vi "FTW-ActorTemplate.vi"(0 "FTW Actor Instance Configuration":string="{\n  \"Identity\": \"ActorName\",\n  \"InboxAddress\": \"inproc://*\",\n  \"PublisherAddress\": \"\",\n  \"LoggerAddress\": \"\",\n  \"DebugEnableInboxLogging\": false,\n  \"DebugEnableJobLogging\": false,\n  \"LauncherAddress\": \"\"\n}", 11 "ErrorIn":errorcluster) -> (15 "Error":errorcluster)   [LabVIEW 2013]
uses:
  src/Instance/FTW-ActorInstance.lvclass
  src/Message/Base/FTW-Message.lvclass
  src/Instance/FTW-ActorInstance.lvclass/FTW-ActorInstance.ctl
  src/JobSequencer/FTW-SEQ-Current.vi
  src/Message/Request/FTW-Message-IncomingRequest.lvclass
panel:
  # "Inputs"
  # "Outputs"
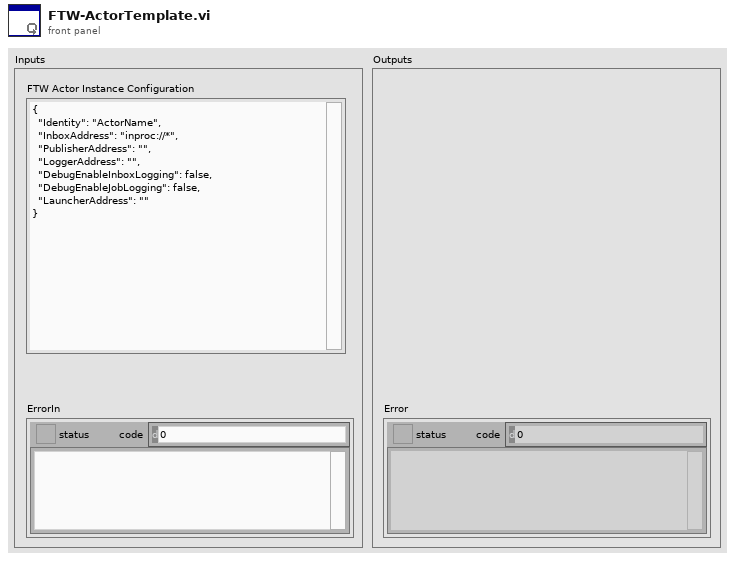
[diagram p1: front panel]
types:
  T1 = cluster{"Incoming Requests":refnum<event-registration>, "Local Messages":refnum<event-registration>, "Additional Registration Types":refnum<event-registration>}
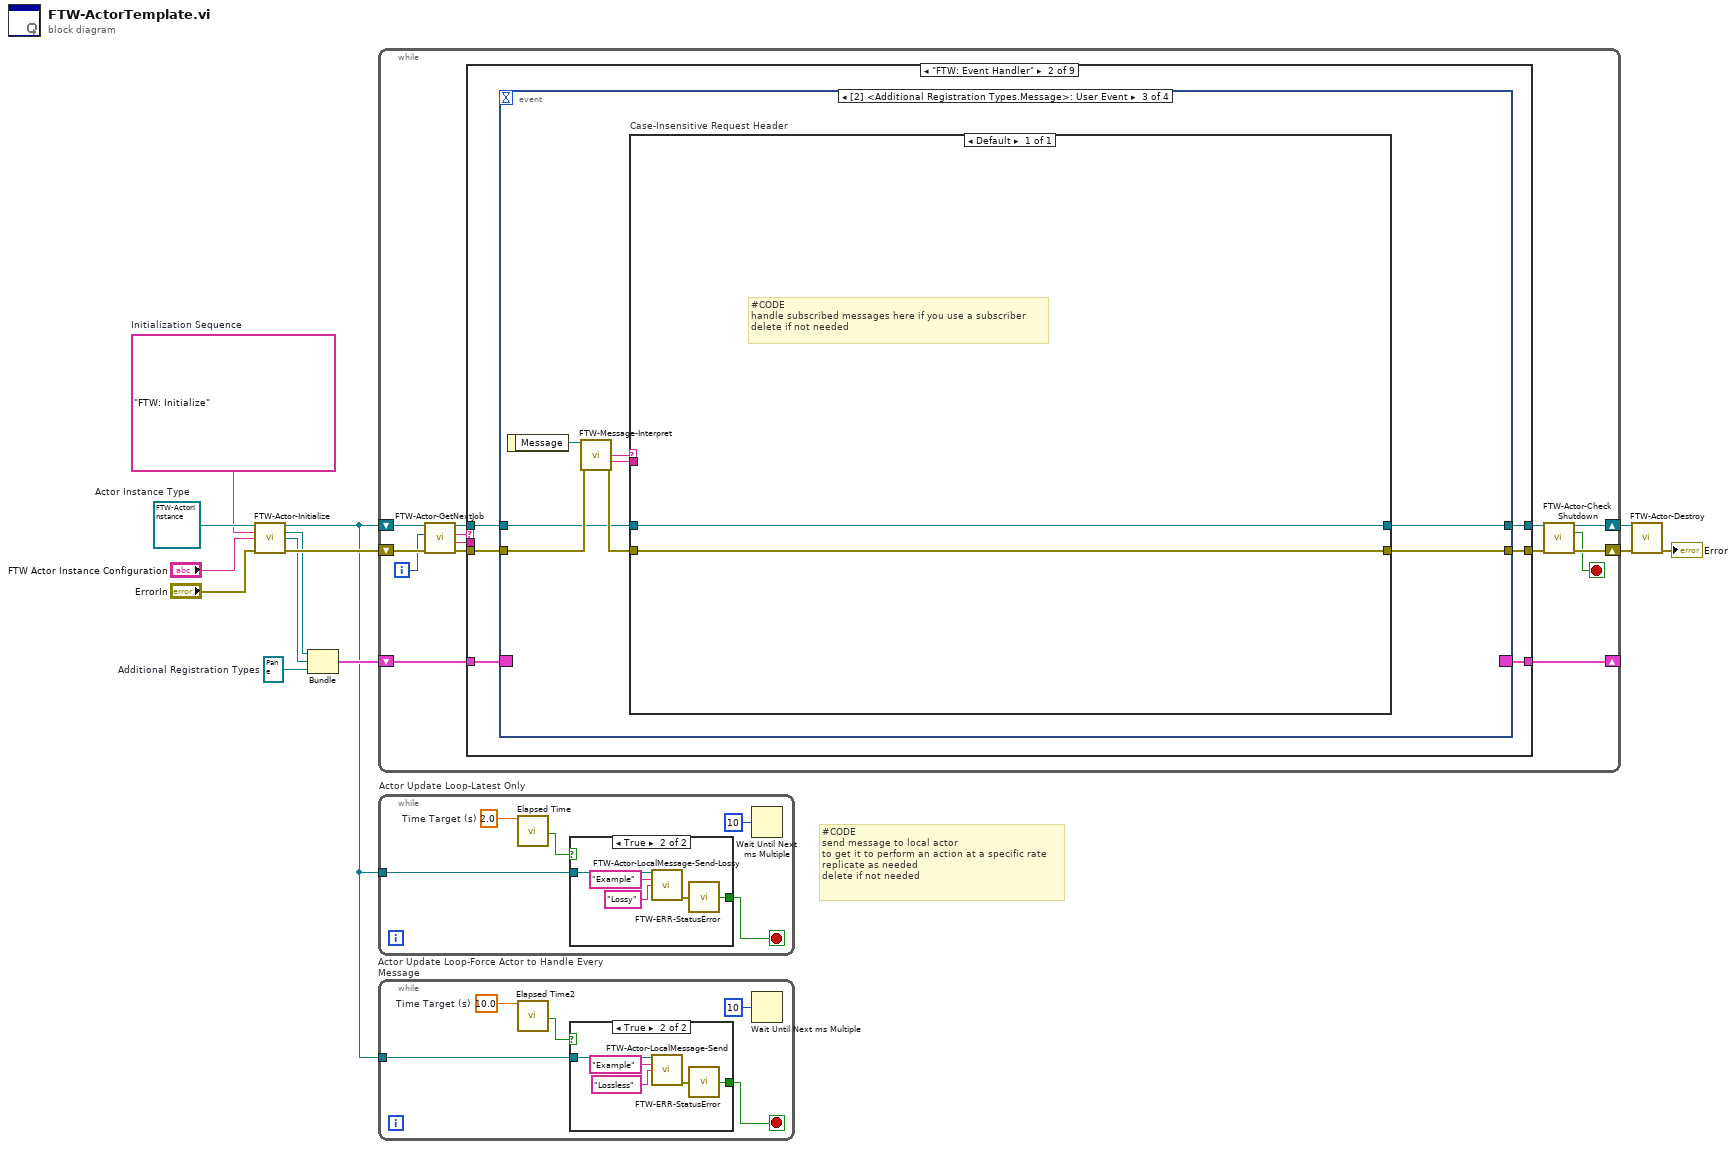
[diagram p0: block diagram]
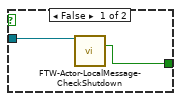
[diagram p2: hidden frame]
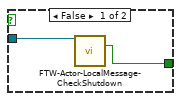
[diagram p3: hidden frame]
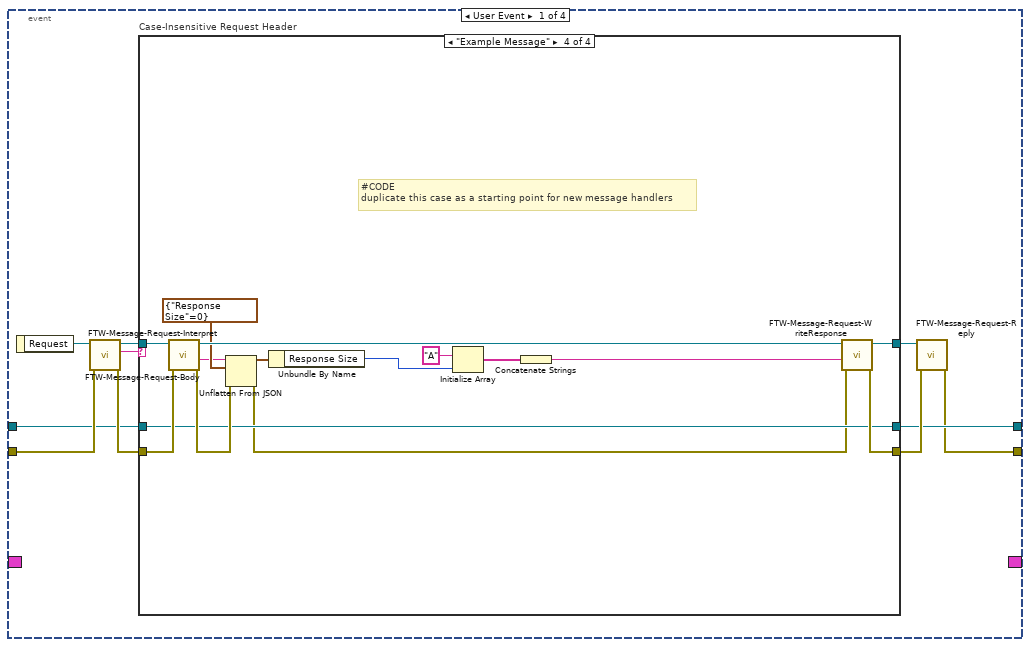
[diagram p5: hidden frame]
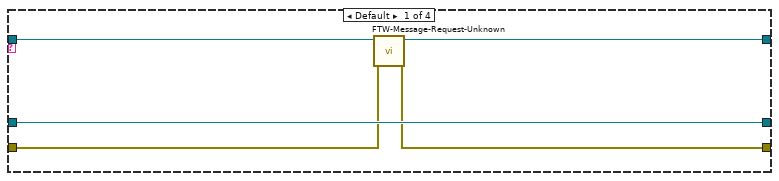
[diagram p6: hidden frame]
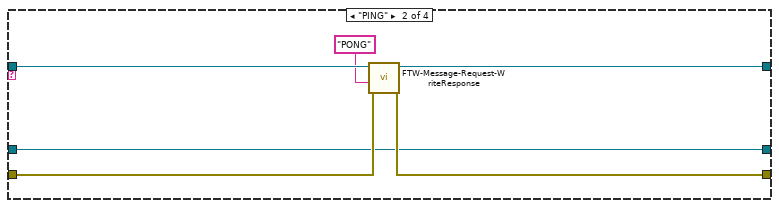
[diagram p7: hidden frame]
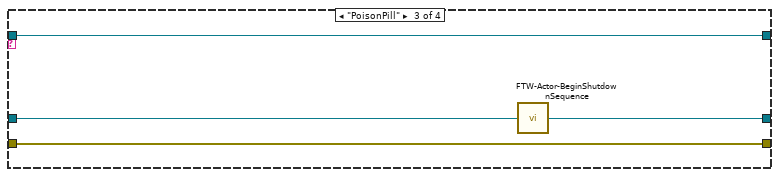
[diagram p8: hidden frame]
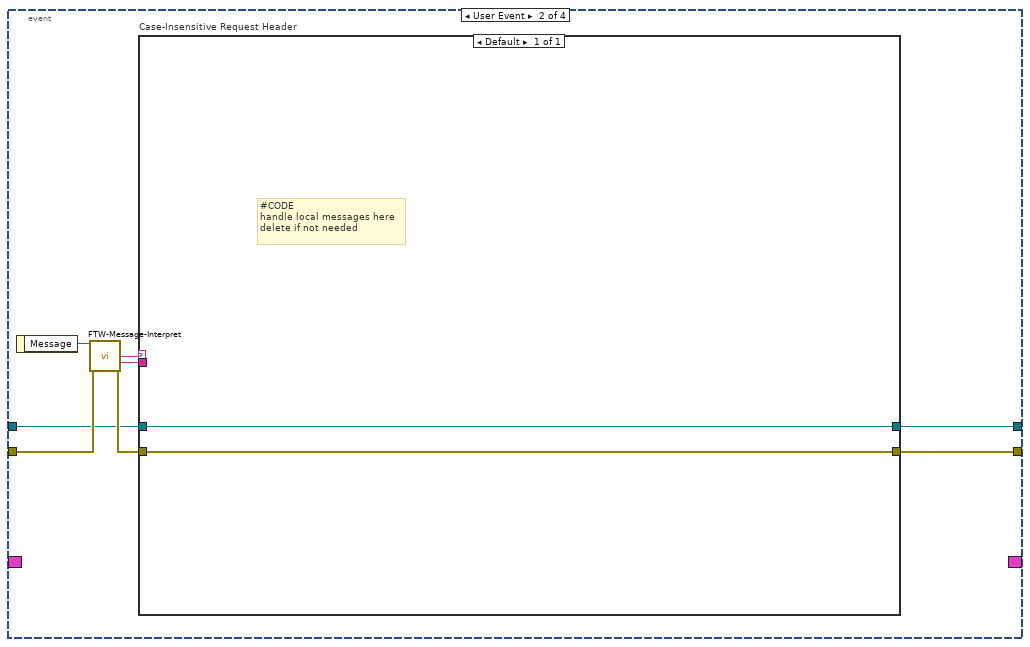
[diagram p9: hidden frame]
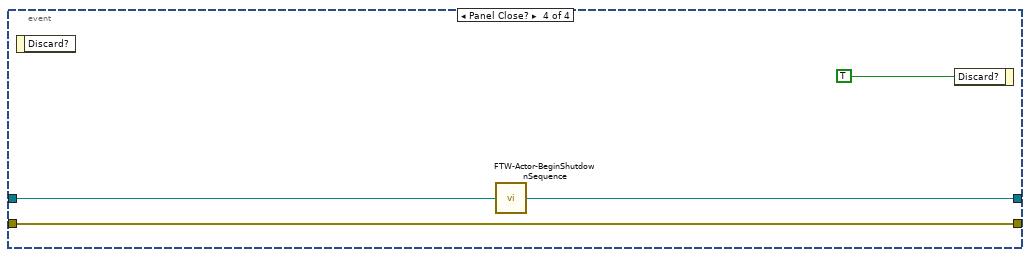
[diagram p10: hidden frame]
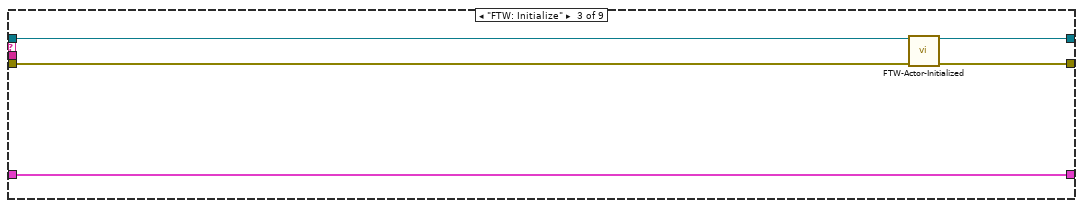
[diagram p11: hidden frame]
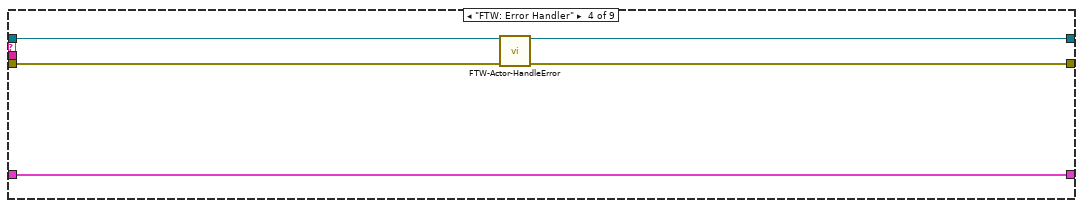
[diagram p12: hidden frame]
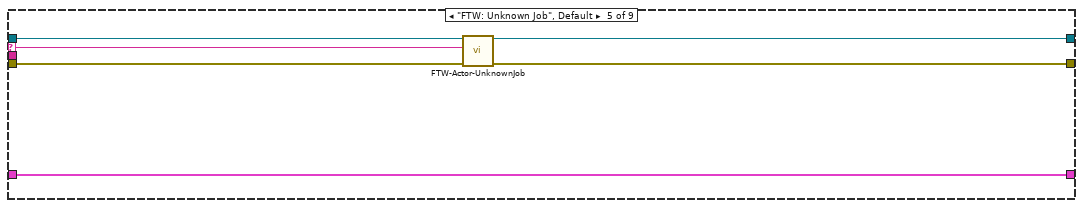
[diagram p13: hidden frame]
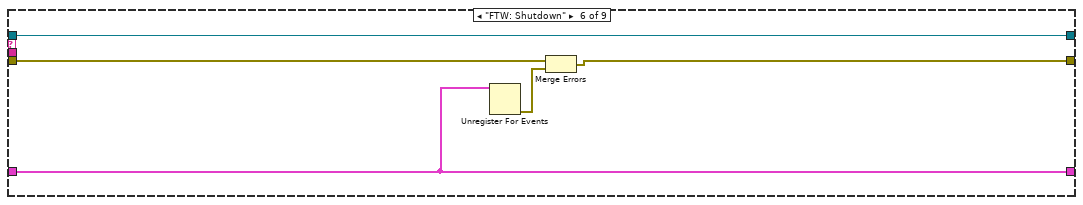
[diagram p14: hidden frame]
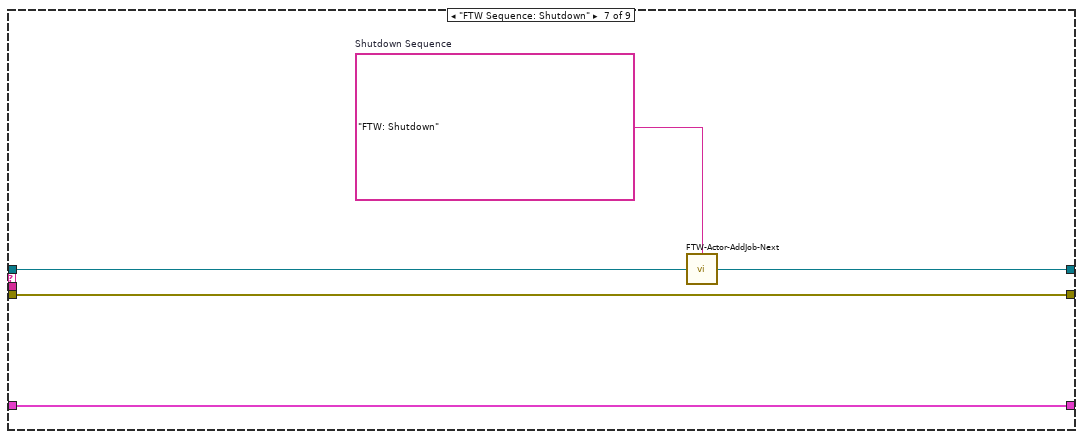
[diagram p15: hidden frame]
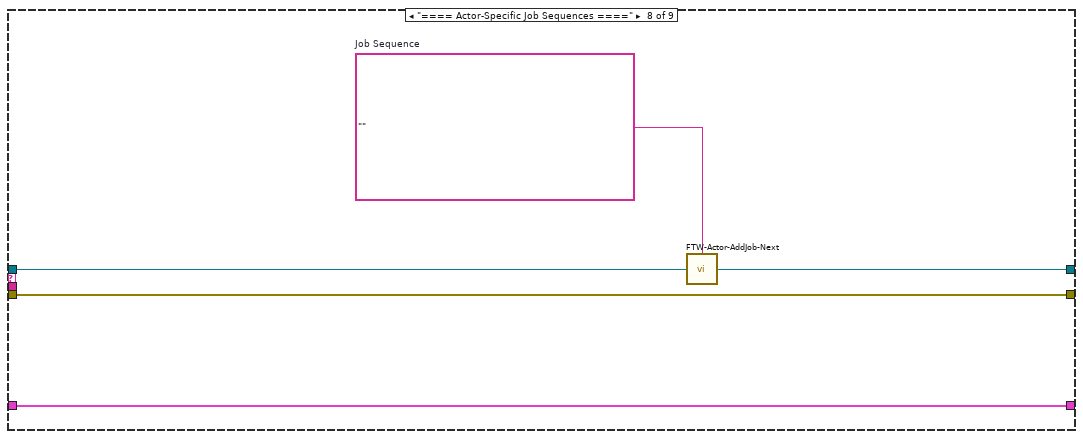
[diagram p16: hidden frame]
diagram:
  w1 = refnum<event-registration> refnum  # Additional Registration Types
  w9 = refnum<class "FTW-ActorInstance.lvclass"> refnum  # Actor Instance Type
  w8 = "FTW: Initialize"  # Initialization Sequence
  # "#CODE\nsend message to local actor\nto get it to perform an action at a specific rate\nreplicate as needed\ndelete if not needed"
  n1 = call-dynamic "FTW-Actor-Initialize.vi"("FTW Actor Instance Type"=w9, "Initialization Job Sequence"=w8, "Actor Instance Configuration"="FTW Actor Instance Configuration", "error in"="ErrorIn") -> ("FTW Actor Instance"=w2:refnum<class "FTW-ActorInstance.lvclass">, "Incoming Requests"=w4:refnum<event-registration>, "Local Messages"=w3:refnum<event-registration>, "error out"=w10:errorcluster)  [unwired: 8 in]
  n2 = Bundle("Incoming Requests"=w4, "Local Messages"=w3, "Additional Registration Types"=w1) -> (w6:T1)  [unwired: 1 in]
  n3 = while {
    shift-right: [w17] -> w12
    shift-left: w10 -> [w24]
    shift-right: [w14] -> _
    shift-left: w6 -> [w27]
    shift-right: [w19] -> w13
    shift-left: w2 -> [w26]
    i -> [w15]
    stop <- w16 stop-if-true
    n4 = call "FTW-Actor-GetNextJob.vi"("error in"=w24, "Jobs Performed"=w15, "FTW Actor Instance"=w26) -> ("error out"=w23:errorcluster, "Job Data"=w21:string, "Job Name"=w22:string, "FTW Actor Instance out"=w25:refnum<class "FTW-ActorInstance.lvclass">)  [unwired: 5 in]
    n5 = case shown="\"FTW: Event Handler\"" w22 {
      selector: w22 -> [_ _ _ _ w111 _ _ _ _]
      tunnel: [w29 w36 w101 w106 w114 w120 w125 w130 w134] -> w18
      tunnel: w23 -> [w29 w35 w104 w108 w115 w121 w125 w130 w134]
      tunnel: w27 -> [w30 w31 w105 w110 w116 w117 w126 w131 w133]
      tunnel: [w30 w34 w105 w110 w116 w117 w126 w131 w133] -> w14
      tunnel: w21 -> [_ _ _ _ _ _ _ _ _]
      tunnel: [w28 w33 w102 w107 w112 w118 w123 w128 w132] -> w20
      tunnel: w25 -> [w28 w32 w103 w109 w113 w118 w124 w129 w132]
      frame "==== Featherweight Framework Jobs ====" {
      }
      frame "FTW: Event Handler" {
        n6 = event shown="[2] <Additional Registration Types.Message>: User Event" {
          selector: w31 -> [_ _ _ _]
          dyn-events: [_ _ _ _] -> w34
          timeout: _ -> [_ _ _ _]
          tunnel: [w38 w81 w91 w99] -> w36
          tunnel: w35 -> [w44 w82 w92 w99]
          tunnel: [w42 w80 w90 w97] -> w33
          tunnel: w32 -> [w41 w79 w89 w98]
          event User Event {
            n7 = event-data() -> ("Request"=w45:refnum<class "FTW-Message-IncomingRequest.lvclass">)  [unwired: 1 in]
            n8 = call "FTW-Message-Request-Interpret.vi"("error in"=w44, "FTW Incoming Request"=w45) -> ("error out"=w46:errorcluster, "Request Header"=w40:string, "FTW Incoming Request out"=w39:refnum<class "FTW-Message-IncomingRequest.lvclass">)  [unwired: 7 in]
            n9 = case "Case-Insensitive Request Header" shown="\"Example Message\"" w40 {
              tunnel: [w49 w55 w60 w73] -> w43
              tunnel: w46 -> [w50 w56 w60 w76]
              tunnel: [w51 w54 w61 w70] -> w42
              tunnel: w41 -> [w51 w54 w59 w70]
              tunnel: w39 -> [w48 w57 w58 w74]
              tunnel: [w47 w53 w58 w71] -> w37
              frame Default {
                n10 = call "FTW-Message-Request-Unknown.vi"("error in"=w50, "FTW Incoming Request"=w48) -> ("error out"=w49:errorcluster, "FTW Incoming Request Out"=w47:refnum<class "FTW-Message-IncomingRequest.lvclass">)  [unwired: 8 in]
              }
              frame "PING" {
                n11 = call "FTW-Message-Request-WriteResponse.vi"("error in"=w56, "Response Body"="PONG" ("Response Header"), "FTW Incoming Request"=w57) -> ("error out"=w55:errorcluster, "FTW Incoming Request out"=w53:refnum<class "FTW-Message-IncomingRequest.lvclass">)  [unwired: 7 in]
              }
              frame "PoisonPill" {
                n12 = call "FTW-Actor-BeginShutdownSequence.vi"("FTW Actor Instance"=w59) -> ("FTW Actor Instance out"=w61:refnum<class "FTW-ActorInstance.lvclass">)  [unwired: 3 in]
              }
              frame "Example Message" {
                # "#CODE\nduplicate this case as a starting point for new message handlers"
                n13 = call "FTW-Message-Request-Body.vi"("error in"=w76, "FTW Incoming Request"=w74) -> ("error out"=w75:errorcluster, "Request Body"=w67:string, "FTW Incoming Request out"=w72:refnum<class "FTW-Message-IncomingRequest.lvclass">)  [unwired: 7 in]
                n14 = Unflatten From JSON(JSON string=w67, type and defaults=cluster{"Response Size":i32} {"Response Size"=0}, error in (no error)=w75) -> (value=w66:cluster{"Response Size":i32}, error out=w69:errorcluster)  [unwired: 4 in]
                n15 = Unbundle By Name(w66) -> ("Response Size"=w65:i32)
                n16 = Initialize Array("A", w65) -> (w63:string[])
                n17 = Concatenate Strings(w63) -> (w62:string)
                n18 = call "FTW-Message-Request-WriteResponse.vi"("error in"=w69, "Response Body"=w62, "FTW Incoming Request"=w72) -> ("error out"=w73:errorcluster, "FTW Incoming Request out"=w71:refnum<class "FTW-Message-IncomingRequest.lvclass">)  [unwired: 7 in]
              }
            }
            n19 = call "FTW-Message-Request-Reply.vi"("error in"=w43, "FTW Incoming Request"=w37) -> ("error out"=w38:errorcluster)  [unwired: 8 in, 1 out]
          }
          event User Event {
            n20 = event-data() -> ("Message"=w83:refnum<class "FTW-Message.lvclass">)  [unwired: 1 in]
            n21 = call-dynamic "FTW-Message-Interpret.vi"("FTW Message"=w83, "error in"=w82) -> ("Message Header"=w77:string, "Message Body"=w78:string, "error out"=w84:errorcluster)  [unwired: 9 in, 2 out]
            n22 = case "Case-Insensitive Request Header" shown="Default" w77 {
              tunnel: [w85] -> w81
              tunnel: w84 -> [w85]
              tunnel: [w86] -> w80
              tunnel: w79 -> [w86]
              tunnel: w78 -> [_]
              frame Default {
                # "#CODE\nhandle local messages here\ndelete if not needed"
              }
            }
          }
          event User Event {
            n23 = event-data() -> ("Message"=w93:refnum<class "FTW-Message.lvclass">)  [unwired: 1 in]
            n24 = call-dynamic "FTW-Message-Interpret.vi"("FTW Message"=w93, "error in"=w92) -> ("Message Header"=w87:string, "Message Body"=w88:string, "error out"=w94:errorcluster)  [unwired: 9 in, 2 out]
            n25 = case "Case-Insensitive Request Header" shown="Default" w87 {
              tunnel: [w95] -> w91
              tunnel: w94 -> [w95]
              tunnel: [w96] -> w90
              tunnel: w89 -> [w96]
              tunnel: w88 -> [_]
              frame Default {
                # "#CODE\nhandle subscribed messages here if you use a subscriber\ndelete if not needed"
              }
            }
          }
          event Panel Close? {
            n26 = event-data() -> ()  [unwired: 1 in, 1 out]
            n27 = call "FTW-Actor-BeginShutdownSequence.vi"("FTW Actor Instance"=w98) -> ("FTW Actor Instance out"=w97:refnum<class "FTW-ActorInstance.lvclass">)  [unwired: 3 in]
            n28 = event-data("Discard?"=TRUE) -> ()  [unwired: 1 in, 1 out]
          }
        }
      }
      frame "FTW: Initialize" {
        n29 = call-dynamic "FTW-Actor-Initialized.vi"("FTW Actor Instance"=w103, "error in"=w104) -> ("FTW Actor Instance out"=w102:refnum<class "FTW-ActorInstance.lvclass">, "error out"=w101:errorcluster)  [unwired: 12 in]
      }
      frame "FTW: Error Handler" {
        n30 = call-dynamic "FTW-Actor-HandleError.vi"("FTW Actor Instance"=w109, "error in"=w108) -> ("FTW Actor Instance out"=w107:refnum<class "FTW-ActorInstance.lvclass">, "error out"=w106:errorcluster)  [unwired: 11 in, 1 out]
      }
      frame "FTW: Unknown Job", Default {
        n31 = call-dynamic "FTW-Actor-UnknownJob.vi"("FTW Actor Instance"=w113, "Unknown Job"=w111, "error in"=w115) -> ("FTW Actor Instance out"=w112:refnum<class "FTW-ActorInstance.lvclass">, "error out"=w114:errorcluster)  [unwired: 11 in]
      }
      frame "FTW: Shutdown" {
        n32 = Unregister For Events(event registration refnum=w117) -> (error out=w119:errorcluster)  [unwired: 1 in]
        n33 = Merge Errors(w121, w119) -> (w120:errorcluster)
      }
      frame "FTW Sequence: Shutdown" {
        w122 = "FTW: Shutdown"  # Shutdown Sequence
        n34 = call "FTW-Actor-AddJob-Next.vi"("Add Next in Job Queue"=w122, "FTW Actor Instance"=w124) -> ("FTW Actor Instance out"=w123:refnum<class "FTW-ActorInstance.lvclass">)  [unwired: 2 in]
      }
      frame "==== Actor-Specific Job Sequences ====" {
        w127 = ""  # Job Sequence
        n35 = call "FTW-Actor-AddJob-Next.vi"("Add Next in Job Queue"=w127, "FTW Actor Instance"=w129) -> ("FTW Actor Instance out"=w128:refnum<class "FTW-ActorInstance.lvclass">)  [unwired: 2 in]
      }
      frame "==== Actor-Specific Jobs ====" {
      }
    }
    n36 = call "FTW-Actor-CheckShutdown.vi"("FTW Actor Instance"=w20, "error in"=w18) -> ("FTW Actor Instance out"=w19:refnum<class "FTW-ActorInstance.lvclass">, "Shutdown?"=w16:bool, "error out"=w17:errorcluster)  [unwired: 11 in]
  }
  n37 = while "Actor Update Loop-Latest Only" {
    tunnel: w2 -> [w139]
    stop <- w138 stop-if-true
    w137 = 2.0  # Time Target (s)
    n38 = call "Elapsed Time"("Time Target (s)"=w137) -> ("Time has Elapsed"=w135:bool)  [unwired: 11 in, 7 out]
    n39 = case shown="True" w135 {
      tunnel: w139 -> [w141 w146]
      tunnel: [w140 w142] -> w138
      frame False {
        n40 = call-dynamic "FTW-Actor-LocalMessage-CheckShutdown.vi"("FTW-ActorInstance In"=w141) -> ("Shutdown"=w140:bool)  [unwired: 14 in]
      }
      frame True {
        n41 = call-dynamic "FTW-Actor-LocalMessage-Send-Lossy.vi"("FTW-ActorInstance In"=w146, "Message Header"="Example", "Message Body"="Lossy") -> ("error out"=w145:errorcluster)  [unwired: 12 in]
        n42 = call "FTW-ERR-StatusError.vi"("error to check"=w145) -> ("Error?"=w142:bool)
      }
    }
    n43 = Wait Until Next ms Multiple(millisecond multiple=u32 10) -> ()  [unwired: 1 out]
  }
  n44 = while "Actor Update Loop-Force Actor to Handle Every Message" {
    tunnel: w2 -> [w151]
    stop <- w150 stop-if-true
    w149 = 10.0  # Time Target (s)
    n45 = call "Elapsed Time2"("Time Target (s)"=w149) -> ("Time has Elapsed"=w147:bool)  [unwired: 11 in, 7 out]
    n46 = case shown="True" w147 {
      tunnel: w151 -> [w153 w158]
      tunnel: [w152 w154] -> w150
      frame False {
        n47 = call-dynamic "FTW-Actor-LocalMessage-CheckShutdown.vi"("FTW-ActorInstance In"=w153) -> ("Shutdown"=w152:bool)  [unwired: 14 in]
      }
      frame True {
        n48 = call-dynamic "FTW-Actor-LocalMessage-Send.vi"("FTW-ActorInstance In"=w158, "Message Header"="Example", "Message Body"="Lossless") -> ("error out"=w157:errorcluster)  [unwired: 12 in]
        n49 = call "FTW-ERR-StatusError.vi"("error to check"=w157) -> ("Error?"=w154:bool)
      }
    }
    n50 = Wait Until Next ms Multiple(millisecond multiple=u32 10) -> ()  [unwired: 1 out]
  }
  n51 = call-dynamic "FTW-Actor-Destroy.vi"("FTW Actor Instance"=w13, "error in"=w12) -> ("error out"=→"Error":errorcluster)  [unwired: 13 in]
